vi "ClientGUIBasique.vi"() -> ()   [LabVIEW 2021]
doc: "Le protocole UDP diffère du protocole TCP car il n'y a pas de détection d'erreur avec les paquets d'informations qui sont envoyés ; il n'y a donc aucune garantie qu'un destinataire reçoive bien des données.\n\nLe protocole UDP offre la possibilité de diffuser des données sur un réseau. Spécifiez simplement une adresse IP de uns (255.255.255.255) pour essayer de diffuser l'information sur tout le réseau. Gardez à l'esprit que des routeurs et d'autres périphériques de réseau refusent généralement de diffuser au-delà de certains points, la diffusion est donc limitée dans la pratique."
panel:
  out "?":u16
  in  "Période\n(en ms)":u32(slide)=100 min=5 max=100 step=5 scale=5.0..100.0
  in  "Instruction\n[1] Get Analog\n[2] Set Digital (PWM)":u8=1 min=1 max=2
  in  "Value [0 - 255]":u8=1
  in  "Pin [0 - 11]":u8=1 max=11
  out "Request Command":u8[](array[numeric])
  out "Response Command":u8[](array[numeric])
  in  "?":bool
  # "Version"
  # "Version"
  # "Instruction"
  # "Argument[0]"
  # "Argument[1]"
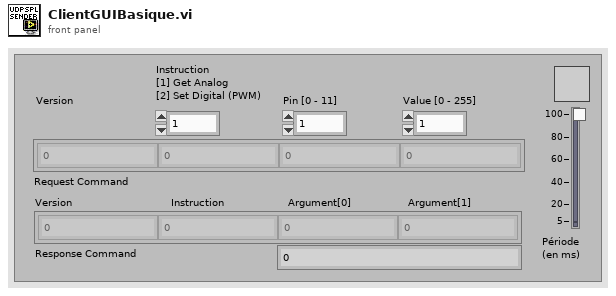
[diagram p1: front panel]
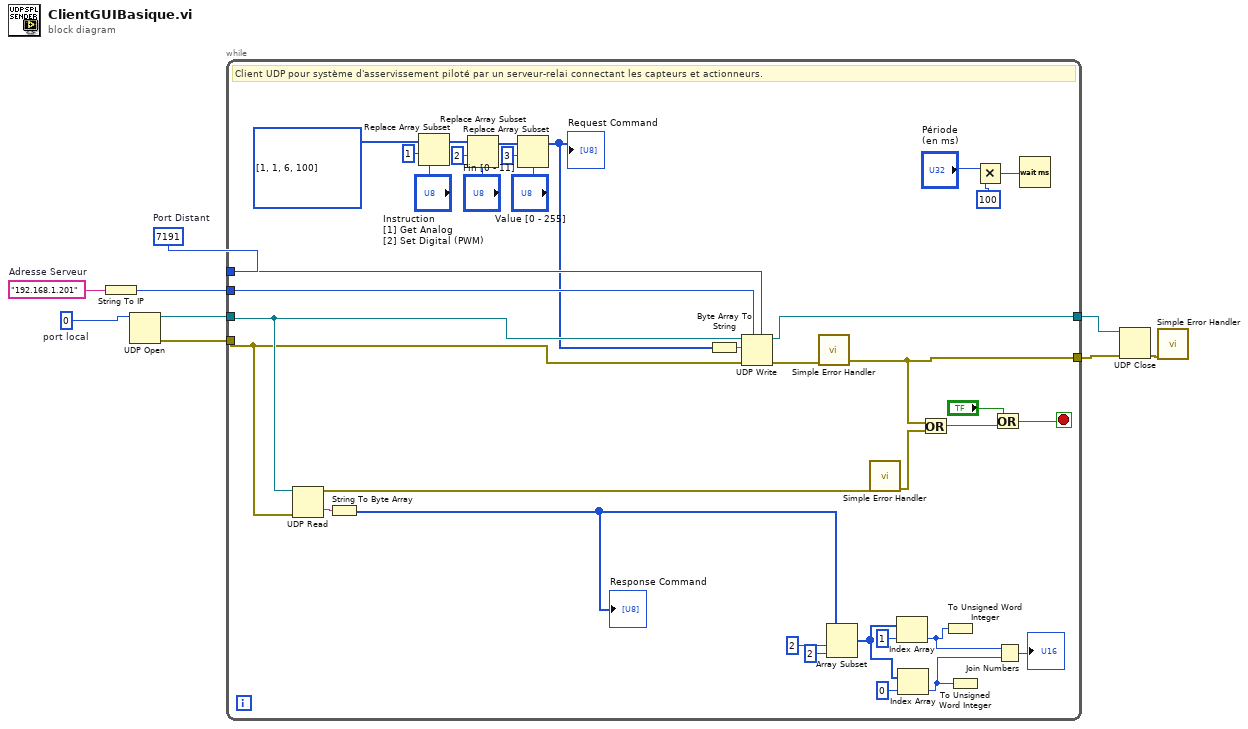
[diagram p0: block diagram]
diagram:
  w2 = u16 7191  # Port Distant
  w6 = u16 0  # port local
  w9 = "192.168.1.201"  # Adresse Serveur
  n1 = String To IP(1:w9) -> (0:w1:u32)
  n2 = UDP Open(11:w6) -> (port=w8:refnum<k16>, 0:w7:errorcluster)  [unwired: 4 in, 1 out]
  n3 = while {
    tunnel: w8 -> [w43]
    tunnel: w7 -> [w33]
    tunnel: w2 -> [w45]
    tunnel: [w28] -> w5
    tunnel: [w27] -> w4
    tunnel: w1 -> [w25]
    stop <- w26 stop-if-true
    # "Client UDP pour système d'asservissement piloté par un serveur-relai connectant les capteurs et actionneurs."
    n4 = UDP Read(connection ID=w43, 8:w33) -> (data out=w42:string, error out=w24:errorcluster)  [unwired: 2 in, 3 out]
    n5 = String To Byte Array(string=w42) -> (unsigned byte array=w13:u8[])
    "Response Command" <- w13
    n6 = Replace Array Subset(array=u8[] [1, 1, 6, 100], new element="Instruction\n[1] Get Analog\n[2] Set Digital (PWM)", index=1 ("indice")) -> (w19:u8[])
    n7 = Replace Array Subset(array=w19, new element="Pin [0 - 11]", index=2 ("indice")) -> (w18:u8[])
    n8 = Replace Array Subset(array=w18, new element="Value [0 - 255]", index=3 ("indice")) -> (w14:u8[])
    "Request Command" <- w14
    n9 = Byte Array To String(unsigned byte array=w14) -> (string=w44:string)
    n10 = UDP Write(address=w25, port or service name=w45, connection ID=w43, data in=w44, 8:w33) -> (error out=w30:errorcluster, 3:w27:refnum<k16>)  [unwired: 1 in]
    n11 = call <vilib>:"Simple Error Handler.vi"(9:w30) -> (6:w28:errorcluster)  [unwired: 4 in, 4 out]
    n12 = Array Subset(array=w13, index=2 ("indice"), length=2 ("longueur")) -> (w37:u8[])
    n13 = call <vilib>:"Simple Error Handler.vi"(9:w24) -> (6:w23:errorcluster)  [unwired: 4 in, 4 out]
    n14 = Index Array(array=w37, index=1 ("indice")) -> (element=w36:u8)
    n15 = Index Array(array=w37, index=0 ("indice")) -> (element=w35:u8)
    n16 = Or(x=w28, y=w23) -> (x .or. y?=w32:bool)
    n17 = To Unsigned Word Integer(number=w36) -> ()  [unwired: 1 out]
    n18 = To Unsigned Word Integer(number=w35) -> ()  [unwired: 1 out]
    n19 = Multiply(x="Période\n(en ms)", y=u32 100) -> (x*y=w12:u32)
    n20 = Or(x="?", y=w32) -> (x .or. y?=w26:bool)
    n21 = Join Numbers(hi=w36, lo=w35) -> ((hi.lo)=→"?":u16)
    n22 = Wait (ms)(milliseconds to wait=w12) -> ()  [unwired: 1 out]
  }
  n23 = UDP Close(connection ID=w4, 8:w5) -> (error out=w3:errorcluster)  [unwired: 1 out]
  n24 = call <vilib>:"Simple Error Handler.vi"(9:w3) -> ()  [unwired: 4 in, 5 out]
